vi "Read Image File Directory.vi"(3 "Litt/BigEnd":bool, 4 "Im_File_Dir Offs":i32, 5 "Image Data in":u8[](array[numeric])) -> (1 "Directories":cluster{"Tags":T1[]}[](array[cluster]), 2 "Image Data out":u8[](array[numeric]))   [LabVIEW 2013, in "Tiff reader.lvlib"]
doc: "Reads the tags and associated data in a tiff file byte stream (Image Data in) starting at an offset (Image File Directory Offset) which is determined using the Read Header.vi. Returns an array of clusters containing the tag and location and format of the assocaited data."
uses:
  Tiff reader.lvlib
  IFD Entry.ctl
  FieldTypes.ctl
  U16ToType.vi
panel:
  out "Time elapsed (ms)":u32
  out "size(s)":i32
  out "Array":u32[](array[numeric])
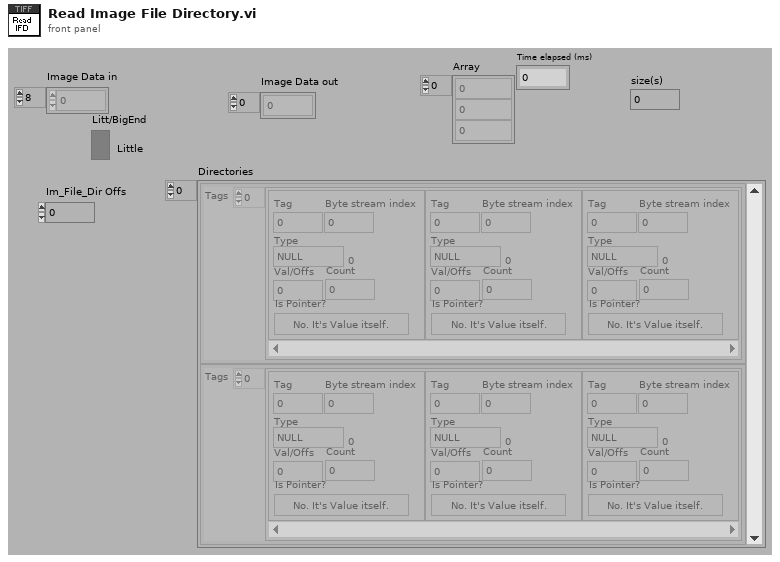
[diagram p1: front panel]
types:
  T1 = typedef "Tiff reader.lvlib/IFD Entry.ctl" = cluster{"Tag":u16, "Type":T2, "Count":u32, "Val/Offs":u32, "Is Pointer?":bool, "Byte stream index":i32}
  T2 = typedef "Tiff reader.lvlib/FieldTypes.ctl" = enum16{"NULL", "U8", "ASCII7", "U16", "U32", "RATIONAL", "SByte(I8)", "Undef(8Bit)", "I16", "I32", "SRat(4B:4B)", "SGL(4Byte)", "DBL(8Byte)"}
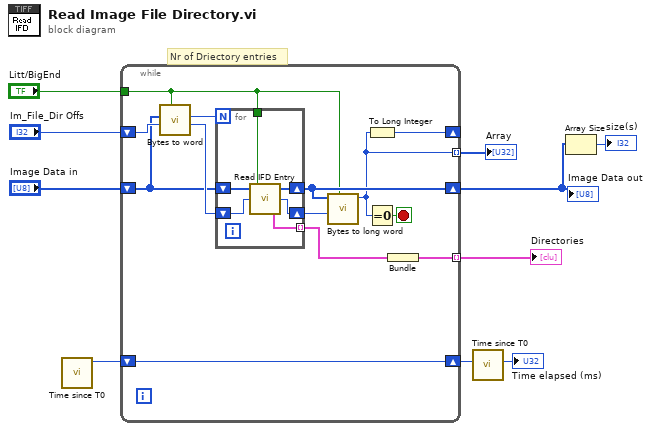
[diagram p0: block diagram]
diagram:
  # "Nr of Driectory entries"
  n1 = call "Time since T0.vi"() -> ("current ms"=w6:u32)  [unwired: 5 in, 2 out]
  n2 = while {
    shift-right: [w18] -> _
    shift-left: "Im_File_Dir Offs" -> [w23]
    tunnel: "Litt/BigEnd" -> [w15]
    tunnel: [w14] -> w8 mode=indexing
    shift-right: [w21] -> w2
    shift-left: "Image Data in" -> [w17]
    shift-right: [w12] -> w5
    shift-left: w6 -> [w12]
    tunnel: [w11] -> w1 mode=indexing
    stop <- w19 stop-if-true
    n3 = call "Bytes to word.vi"("Litt/BigEnd"=w15, "Index"=w23, "Image Data in"=w17) -> ("Index+2"=w22:i32, "Word"=w16:u16)  [unwired: 1 in, 4 out]
    n4 = for {
      N: w16 -> [_]
      shift-right: [w27] -> w21
      shift-left: w17 -> [w28]
      shift-right: [w26] -> w20
      shift-left: w22 -> [w29]
      tunnel: [w25] -> w13 mode=indexing
      tunnel: w15 -> [w24]
      n5 = call "Read IFD Entry.vi"("Litt/BigEnd"=w24, "Directory Offset in"=w29, "Image Data in"=w28) -> ("Cluster"=w25:T1, "Next Directory Offset Out\n(IN + 12)"=w26:i32, "Image Data Out"=w27:u8[])
    }
    n6 = call "Bytes to long word.vi"("Litt/BigEnd"=w15, "Index"=w20, "Image Data in"=w21) -> ("U32"=w14:u32)  [unwired: 6 out]
    n7 = To Long Integer(number=w14) -> (32bit integer=w18:i32)
    n8 = Equal To 0?(x=w14) -> (x = 0?=w19:bool)
    n9 = Bundle(w13) -> (w11:cluster{T1[]})  [unwired: 1 in]
  }
  "Image Data out" <- w2
  "Directories" <- w1
  "Array" <- w8
  n10 = call "Time since T0.vi"("T0 millisecond timer value"=w5) -> ("Time elapsed (ms)"=→"Time elapsed (ms)":u32)  [unwired: 4 in, 2 out]
  n11 = Array Size(array=w2) -> (size(s)=→"size(s)":i32)
